vi "Conv_Centimeters_Meters.vi"(10 "Centimeter":dbl) -> (2 "Meters":dbl)   [LabVIEW 2019, in "Trajectory_Library.lvlib"]
doc: "Convert Centimeters to Meters"
uses:
  Trajectory_Library.lvlib
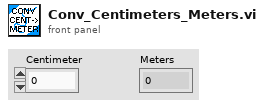
[diagram p1: front panel]
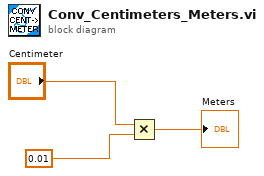
[diagram p0: block diagram]
diagram:
  n1 = Multiply(x="Centimeter", y=0.01) -> (x*y=→"Meters":dbl)
